vi "Untitled 1.vi"() -> ()   [LabVIEW 2015]
panel:
  out "String":string
  out "Счет":u8
  out "Стакан 4":refnum<vi>
  in  "stop":bool
  out "Стакан 3":bool
  out "Стакан 2":bool
  out "Стакан 1":bool
  in  "Играть":bool
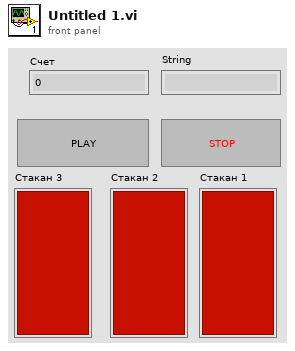
[diagram p1: front panel]
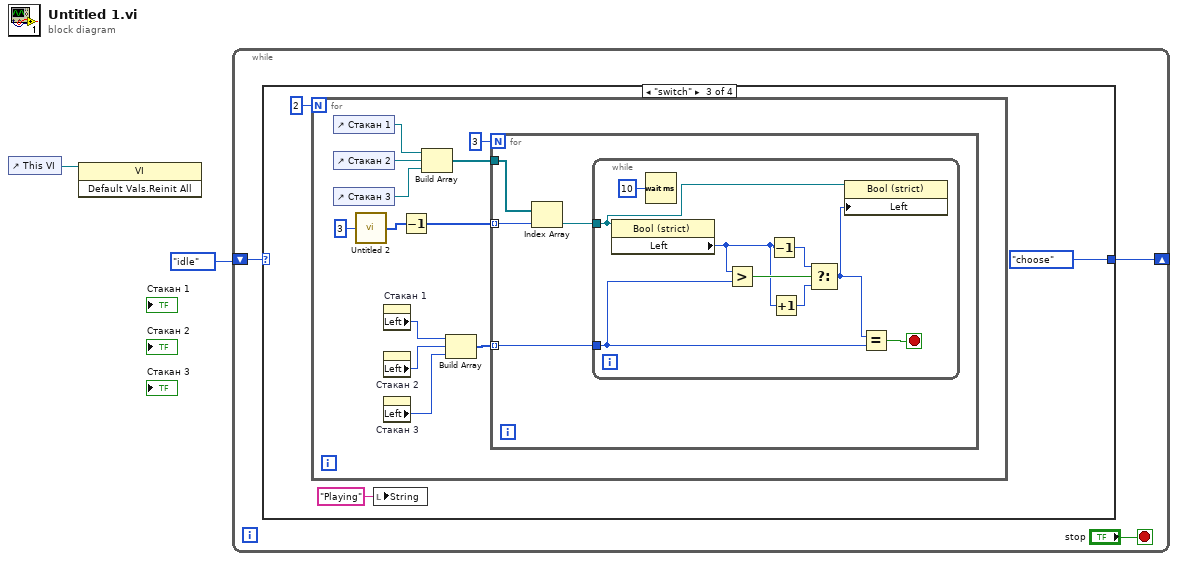
[diagram p0: block diagram]
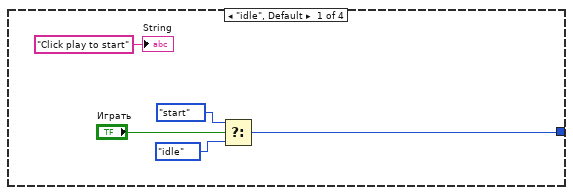
[diagram p2: hidden frame]
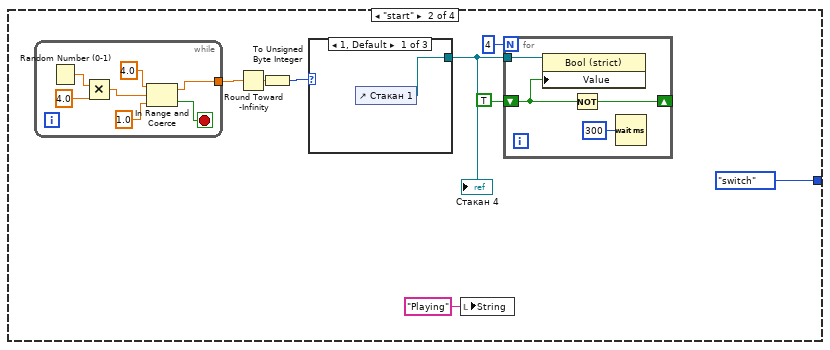
[diagram p3: hidden frame]
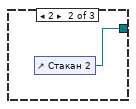
[diagram p4: hidden frame]
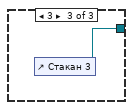
[diagram p5: hidden frame]
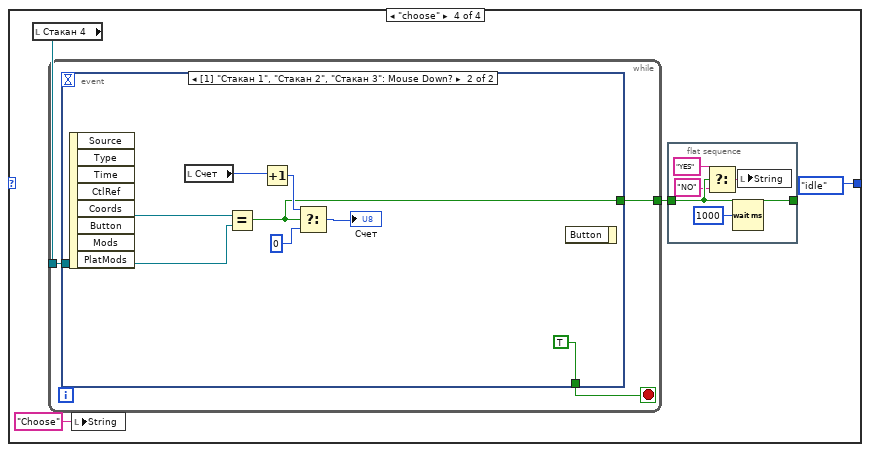
[diagram p6: hidden frame]
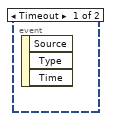
[diagram p7: hidden frame]
diagram:
  n1 = control-ref of="This VI"() -> (w2:refnum<vi>)
  n2 = invoke class="VI" method="Default Vals.Reinit All"(reference=w2) -> ()  [unwired: 2 in, 3 out]
  n3 = while {
    shift-right: [w4] -> _
    shift-left: enum16{"idle", "start", "switch", "choose"}."idle" ("Enum") -> [w5]
    stop <- "stop" stop-if-true
    n4 = case shown="\"switch\"" w5 {
      tunnel: [w7 enum16{"idle", "start", "switch", "choose"}."switch" ("Enum") enum16{"idle", "start", "switch", "choose"}."choose" ("Enum") enum16{"idle", "start", "switch", "choose"}."idle" ("Enum")] -> w4
      frame "idle", Default {
        n5 = Select(t=enum16{"idle", "start", "switch", "choose"}."start" ("Enum"), s="Играть", f=enum16{"idle", "start", "switch", "choose"}."idle" ("Enum")) -> (s? t:f=w7:enum16{"idle", "start", "switch", "choose"})
        "String" <- "Click play to start" ("String")
      }
      frame "start" {
        n6 = while {
          tunnel: [w26] -> w17
          stop <- w30 stop-if-true
          n7 = Random Number (0-1)() -> (number: 0 to 1=w31:dbl)
          n8 = Multiply(x=w31, y=4.0) -> (x*y=w27:dbl)
          n9 = In Range and Coerce(upper limit=4.0, x=w27, lower limit=1.0) -> (coerced(x)=w26:dbl, In Range?=w30:bool)
        }
        n10 = Round Toward -Infinity(1:w17) -> (0:w18:dbl)
        n11 = To Unsigned Byte Integer(number=w18) -> (unsigned 8bit integer=w15:u8)
        n12 = case shown="1, Default" w15 {
          tunnel: [w23 w24 w25] -> w12
          frame 1, Default {
            n13 = control-ref of="Стакан 1"() -> (w23:refnum<vi>)
          }
          frame 2 {
            n14 = control-ref of="Стакан 2"() -> (w24:refnum<vi>)
          }
          frame 3 {
            n15 = control-ref of="Стакан 3"() -> (w25:refnum<vi>)
          }
        }
        "Стакан 4" <- w12
        n16 = local write "String"("Playing" ("String")) -> ()
        n17 = for {
          N: 4 -> [_]
          tunnel: w12 -> [w22]
          shift-right: [w20] -> _
          shift-left: TRUE ("Value") -> [w19]
          n18 = property class="Bool (strict)"(reference=w22, "Value"=w19) -> ()  [unwired: 1 in, 2 out]
          n19 = Not(x=w19) -> (.not. x?=w20:bool)
          n20 = Wait (ms)(milliseconds to wait=u32 300) -> ()  [unwired: 1 out]
        }
      }
      frame "switch" {
        n21 = for {
          N: 2 -> [_]
          n22 = control-ref of="Стакан 1"() -> (w45:refnum<vi>)
          n23 = control-ref of="Стакан 2"() -> (w44:refnum<vi>)
          n24 = control-ref of="Стакан 3"() -> (w43:refnum<vi>)
          n25 = call "Untitled 2.vi"("Numeric"=3) -> ("Array"=w41:i32[])
          n26 = property on="Стакан 1" class="Bool (strict)"() -> ("Left"=w38:i32)  [unwired: 2 in, 2 out]
          n27 = property on="Стакан 2" class="Bool (strict)"() -> ("Left"=w37:i32)  [unwired: 2 in, 2 out]
          n28 = property on="Стакан 3" class="Bool (strict)"() -> ("Left"=w36:i32)  [unwired: 2 in, 2 out]
          n29 = Decrement(x=w41) -> (x-1=w40:i32[])
          n30 = Build Array(w45, w44, w43) -> (w46:refnum<vi>[])
          n31 = Build Array(w38, w37, w36) -> (w39:i32[])
          n32 = for {
            N: 3 -> [_]
            tunnel: w46 -> [w50]
            tunnel: w40 -> [w51] mode=indexing
            tunnel: w39 -> [w48] mode=indexing
            n33 = Index Array(array=w50, index=w51) -> (element=w49:refnum<vi>)
            n34 = while {
              tunnel: w49 -> [w53]
              tunnel: w48 -> [w52]
              stop <- w60 stop-if-true
              n35 = property class="Bool (strict)"(reference=w53) -> ("Left"=w58:i32)  [unwired: 1 in, 2 out]
              n36 = Wait (ms)(milliseconds to wait=u32 10) -> ()  [unwired: 1 out]
              n37 = Greater?(x=w58, y=w52) -> (0:w59:bool)
              n38 = Decrement(x=w58) -> (x-1=w56:i32)
              n39 = Increment(x=w58) -> (x+1=w57:i32)
              n40 = Select(t=w56, s=w59, f=w57) -> (s? t:f=w54:i32)
              n41 = property class="Bool (strict)"(reference=w53, "Left"=w54) -> ()  [unwired: 1 in, 2 out]
              n42 = Equal?(x=w54, y=w52) -> (x = y?=w60:bool)
            }
          }
        }
        n43 = local write "String"("Playing" ("String")) -> ()
      }
      frame "choose" {
        n44 = local read "Стакан 4"() -> (w64:refnum<vi>)
        n45 = while {
          tunnel: w64 -> [w72]
          tunnel: [w70] -> w63
          stop <- w71 stop-if-true
          n46 = event shown="[1] \"Стакан 1\", \"Стакан 2\", \"Стакан 3\": Mouse Down?" {
            selector: _ -> [_ _]
            dyn-events: _ -> [_ _]
            timeout: _ -> [_ _]
            tunnel: w72 -> [_ w79]
            tunnel: [_ TRUE] -> w71
            tunnel: [_ w75] -> w70
            event Timeout {
              n47 = event-data() -> ()  [unwired: 1 in, 3 out]
            }
            event "Стакан 1", "Стакан 2", "Стакан 3": Mouse Down? {
              n48 = event-data() -> ("CtlRef"=w80:refnum<vi>)  [unwired: 1 in, 7 out]
              n49 = local read "Счет"() -> (w74:u8)
              n50 = Equal?(x=w80, y=w79) -> (x = y?=w75:bool)
              n51 = Increment(x=w74) -> (x+1=w77:u8)
              n52 = Select(t=w77, s=w75, f=u8 0) -> (s? t:f=→"Счет":u8)
              n53 = event-data() -> ()  [unwired: 2 in, 1 out]
            }
          }
        }
        n54 = local write "String"("Choose" ("String")) -> ()
        n55 = flat-sequence {
          tunnel: w63 -> [w66]
          tunnel: [w66] -> _
          frame #0 {
            n56 = Select(t="YES", s=w66, f="NO") -> (s? t:f=w69:string)
            n57 = Wait (ms)(milliseconds to wait=u32 1000) -> ()  [unwired: 1 out]
            n58 = local write "String"(w69) -> ()
          }
        }
      }
    }
  }
